vi "Read DBL refnum.vi"(8 "error in (no error)":errorcluster, 11 "DBL Result Class in":refnum<class "DBL Result Class.lvclass">) -> (0 "error out":errorcluster, 2 "DBL refnum":refnum<vi>, 3 "DBL Result Class out":refnum<class "DBL Result Class.lvclass">)   [LabVIEW 2021, in "DBL Result Class.lvclass"]
uses:
  DBL Result Class.lvclass
  DBL Result Class.lvclass/DBL Result Class.ctl
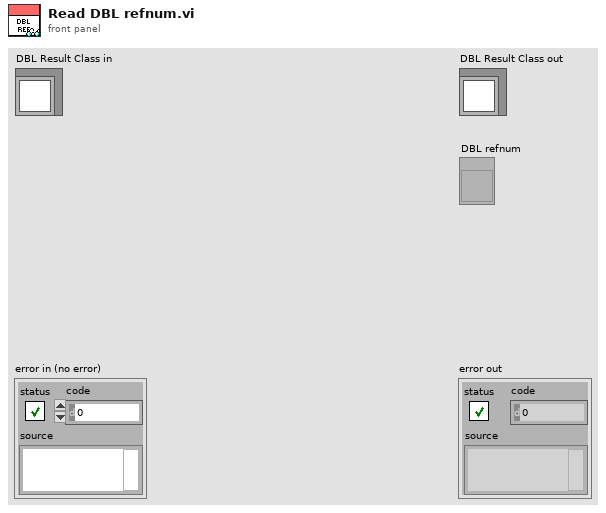
[diagram p1: front panel]
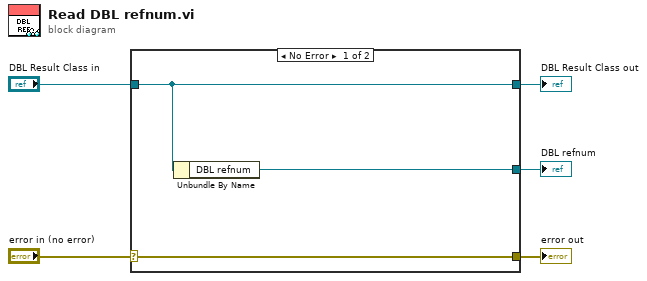
[diagram p0: block diagram]
diagram:
  n1 = case shown="No Error" "error in (no error)" {
    selector: "error in (no error)" -> [w8 w9]
    tunnel: [w8 w9] -> w4
    tunnel: [w7 w10] -> w2
    tunnel: "DBL Result Class in" -> [w7 w10]
    tunnel: [w6 _] -> w1
    frame No Error {
      n2 = Unbundle By Name(w7) -> ("DBL refnum"=w6:refnum<vi>)
    }
    frame Error {
    }
  }
  "error out" <- w4
  "DBL Result Class out" <- w2
  "DBL refnum" <- w1
